vi "429 External PXI Trigger.vi"() -> ()   [LabVIEW 2019]
doc: "This example program configures the Card to transmit a message based \non an external PXI trigger. It also allows the message to be software triggered. The message count is incremented with each transmission of the message and the LED is illuminated.\n\nNote: The message can be triggered externally with a device such as NI-PXIe 6674T that is configured to route the signal to PXI_TRIG[0]. Other trigger lines may be utilized by changing the configuration file."
uses:
  <instrlib>/BTICardLib/Public/Controls/Software Trigger Line Select.ctl
  <instrlib>/BTICardLib/Private/Initialize By Card Number and Core Number.vi
  <instrlib>/BTI429Lib/Private/Tx/Configure/Configure Tx Channel From XML.vi
  <instrlib>/BTI429Lib/Private/Core/Action-Status/Start Channel.vi
  <instrlib>/BTI429Lib/Private/Core/Action-Status/Stop All Channels.vi
  <instrlib>/BTICardLib/BTICardLV.lvlib
  <instrlib>/BTI429Lib/BTI429LV.lvlib
panel:
  in  "Raw Message":u32=2863311530 format="%08x"
  out "Xmit Count":u32
  out "Triggered ?":bool
  out "Error":errorcluster
  in  "Set Message Data":bool
  in  "?":bool
  in  "Software Trigger":bool
  in  "Channel XML Configuration":string="429 External PXI Trigger.xml"
  in  "Card Number":i32
  # "ARINC 429 External PXI Trigger"
  # "©2016 Astronics Ballard Technology"
  # "This example program configures the Card to transmit a message based \non an external PXI trigger. It also allows the message to be software triggered. The message count is incremented with each transmission of the message and the LED is illuminated.\n\nNote: The message can be triggered externally with a device such as NI-PXIe 6674T that is configured to route the  signal to PXI_TRIG[0]. Other trigger lines may be utilized by changing the configuration file."
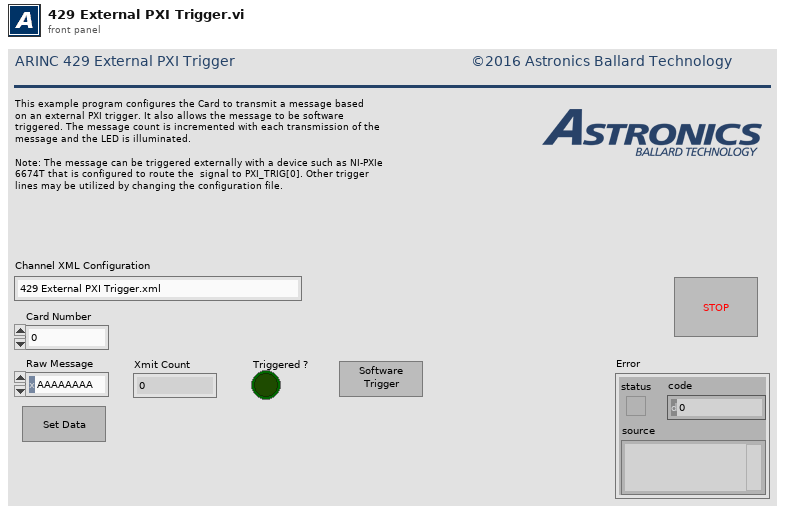
[diagram p1: front panel]
types:
  T1 = typedef "BTICardLV.lvlib/Software Trigger Line Select.ctl" = cluster{"triggerlinea":bool, "triggerlineb":bool, "triggerlinec":bool}
  T2 = typedef "BTI429LV.lvlib/429 Message Fields.ctl" = cluster{"channelnumber":i32, "speed":u32, "gaperror":bool, "parityerror":bool, "longworderror":bool, "bittimeerror":bool, "timeouterror":bool, "reserved":i8, "reserved":i8, "reserved":i8, "anyerror":bool, "hit":bool, "reserved":i8, "reserved":i8, "msgdata":u32, "timetagh":u32, "timetag_hitcount":u32, "maxtime_elapsetime":u32, "mintime":u32, "decgap":u16, "paramflag":u16}
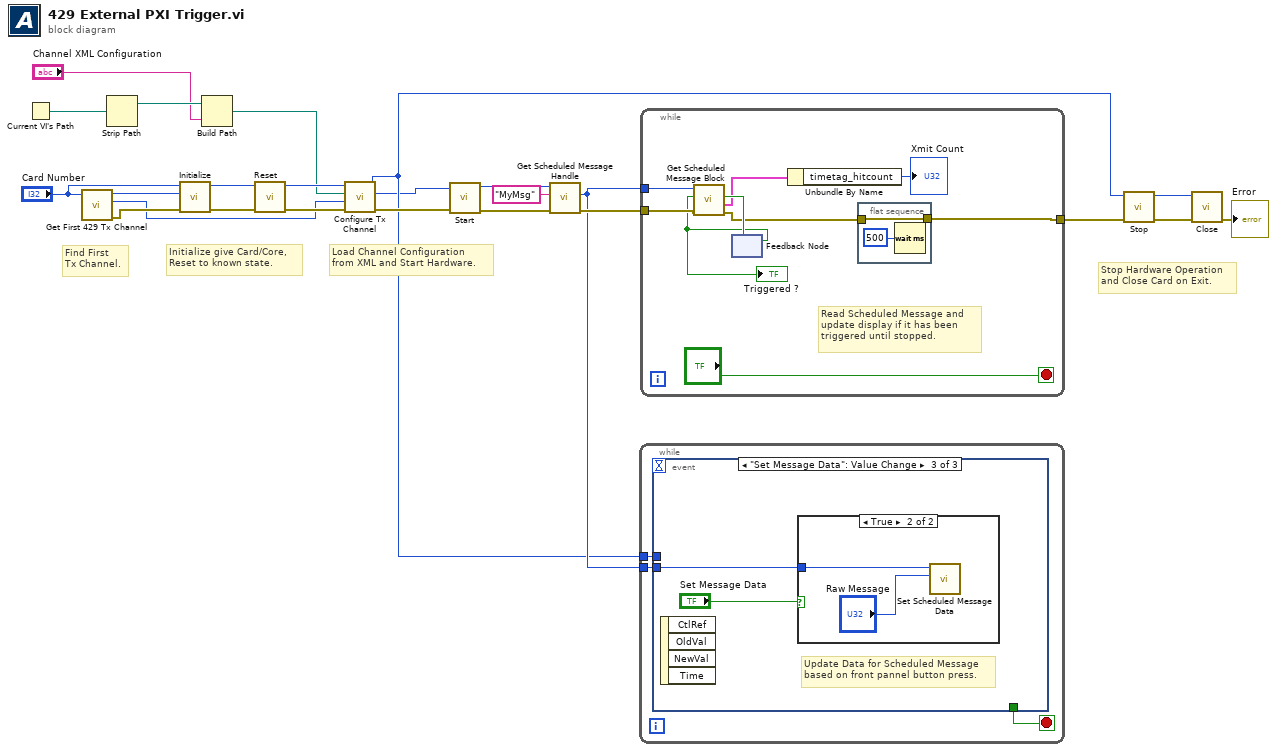
[diagram p0: block diagram]
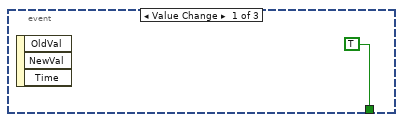
[diagram p2: hidden frame]
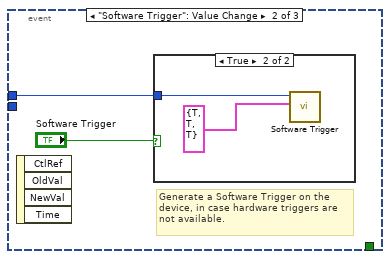
[diagram p3: hidden frame]
diagram:
  # "Stop Hardware Operation\nand Close Card on Exit."
  # "Load Channel Configuration\nfrom XML and Start Hardware."
  # "Initialize give Card/Core, \nReset to known state."
  # "Find First\nTx Channel."
  n1 = Current VI's Path() -> (path=w19:path)
  n2 = call "Get First 429 Tx Channel.vi"("Card Number"="Card Number") -> ("error out"=w21:errorcluster, "Channel Number"=w13:i32, "Core Number"=w23:i32)  [unwired: 8 in]
  n3 = Strip Path(path=w19) -> (stripped path=w18:path)  [unwired: 1 out]
  n4 = call-poly <instrlib>:"Initialize.vi"("error in (no error)"=w21, "core number"=w23, "card number"="Card Number") -> ("error out"=w20:errorcluster, "core handle out"=w24:u64)  [unwired: 7 in]
  n5 = Build Path(base path=w18, name or relative path="Channel XML Configuration") -> (appended path=w14:path)
  n6 = call <instrlib>:"Reset.vi"("error in (no error)"=w20, "core handle in"=w24) -> ("error out"=w16:errorcluster, "core handle out"=w15:u64)  [unwired: 8 in]
  n7 = call-poly <instrlib>:"Configure Tx Channel.vi"("error in (no error)"=w16, "channel number in"=w13, "configuration file path"=w14, "core handle in"=w15) -> ("error out"=w10:errorcluster, "channel handle out"=w1:u64, "core handle out"=w2:u64)  [unwired: 5 in]
  n8 = call-poly <instrlib>:"Start.vi"("error in (no error)"=w10, "channel handle in"=w1) -> ("error out"=w8:errorcluster, "channel handle out"=w9:u64)  [unwired: 8 in]
  n9 = call <instrlib>:"Get Scheduled Message Handle.vi"("error in (no error)"=w8, "message name"="MyMsg", "channel handle in"=w9) -> ("error out"=w6:errorcluster, "message handle out"=w5:u64)  [unwired: 6 in, 1 out]
  n10 = while {
    tunnel: w5 -> [w27]
    tunnel: w2 -> [w26]
    stop <- w25 stop-if-true
    n11 = event shown="[2] \"Set Message Data\": Value Change" {
      selector: _ -> [_ _ _]
      dyn-events: _ -> [_ _ _]
      timeout: _ -> [_ _ _]
      tunnel: [TRUE ("Stop Reading/Writing PXI Signals\nand Close the card") _ _] -> w25
      tunnel: w27 -> [_ _ w33]
      tunnel: w26 -> [_ w29 _]
      event Value Change {
        n12 = event-data() -> ()  [unwired: 1 in, 3 out]
      }
      event "Software Trigger": Value Change {
        # "Generate a Software Trigger on the\ndevice, in case hardware triggers are \nnot available."
        n13 = event-data() -> ()  [unwired: 1 in, 4 out]
        n14 = case shown="True" "Software Trigger" {
          tunnel: w29 -> [_ w32]
          frame False {
          }
          frame True {
            n15 = call <instrlib>:"Software Trigger.vi"("trigger line select"=T1 {"triggerlinea"=TRUE, "triggerlineb"=TRUE, "triggerlinec"=TRUE}, "core handle in"=w32) -> ()  [unwired: 8 in, 2 out]
          }
        }
      }
      event "Set Message Data": Value Change {
        # "Update Data for Scheduled Message\nbased on front pannel button press."
        n16 = event-data() -> ()  [unwired: 1 in, 4 out]
        n17 = case shown="True" "Set Message Data" {
          tunnel: w33 -> [_ w36]
          frame False {
          }
          frame True {
            n18 = call <instrlib>:"Set Scheduled Message Data.vi"("value"="Raw Message", "message handle in"=w36) -> ()  [unwired: 8 in, 2 out]
          }
        }
      }
    }
  }
  n19 = while {
    tunnel: w6 -> [w43]
    tunnel: w5 -> [w44]
    tunnel: [w38] -> w4
    stop <- "?" stop-if-true
    # "Read Scheduled Message and \nupdate display if it has been \ntriggered until stopped."
    n20 = feedback #1() -> (w41:bool)  [unwired: 1 in]
    "Triggered ?" <- w41
    n21 = call <instrlib>:"Get Scheduled Message Block.vi"("error in (no error)"=w43, "clear hit?"=w41, "message handle in"=w44) -> ("error out"=w37:errorcluster, "value"=w40:T2, "was hit?"=w42:bool)  [unwired: 5 in, 1 out]
    n22 = feedback-in #1(w42) -> ()
    n23 = Unbundle By Name(w40) -> ("timetag_hitcount"=→"Xmit Count":u32)
    n24 = flat-sequence {
      tunnel: w37 -> [w46]
      tunnel: [w46] -> w38
      frame #0 {
        n25 = Wait (ms)(milliseconds to wait=u32 500) -> ()  [unwired: 1 out]
      }
    }
  }
  n26 = call-poly <instrlib>:"Stop.vi"("error in (no error)"=w4, "core handle in"=w2) -> ("error out"=w12:errorcluster, "core handle out"=w11:u64)  [unwired: 8 in]
  n27 = call <instrlib>:"Close.vi"("error in (no error)"=w12, "core handle in"=w11) -> ("error out"=→"Error":errorcluster)  [unwired: 8 in, 1 out]
